vi "OA Delete Mode.vi"(10 "uiModeNameLen":u32, 11 "pcModeName":string) -> (3 "function return":u32)   [LabVIEW 2018, in "Copy of Andor SDK.lvlib"]
doc: "EXPNETTYPE unsigned int WINAPI OA_DeleteMode(const char * const pcModeName, unsigned int uiModeNameLen);"
uses:
  Copy of Andor SDK.lvlib
  <userlib>/Andor SDK/ATMCD32D.dll
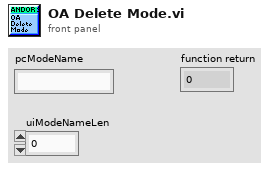
[diagram p1: front panel]
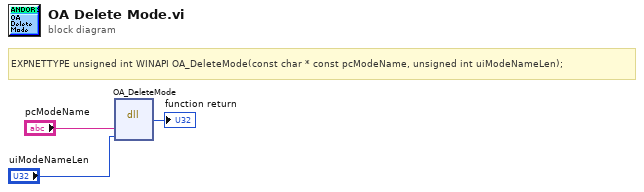
[diagram p0: block diagram]
diagram:
  # "EXPNETTYPE unsigned int WINAPI OA_DeleteMode(const char * const pcModeName, unsigned int uiModeNameLen);"
  n1 = dll-call lib="C:/Program Files (x86)/National Instruments/LabVIEW 2018/user.lib/Andor SDK/ATMCD32D.*" fn="OA_DeleteMode"("pcModeName"="pcModeName", "uiModeNameLen"="uiModeNameLen") -> (→"function return":u32)  [unwired: 5 in, 2 out]
